vi "Test MQTT-2.3.1-5.vi"(8 "error in (no error)":errorcluster) -> (0 "error out":errorcluster)   [LabVIEW 2013]
uses:
  <vilib>/LabVIEW Open Source Project/MQTT Control Packets/Control Packets/ControlPacket/QualityOfService -- enum.ctl
  <vilib>/LabVIEW Open Source Project/MQTT Control Packets/Control Packets/ControlPacket/ControlPacket.lvclass/ControlPacket.ctl
  <vilib>/addons/_JKI Toolkits/Caraya/classes/Test/Test.lvclass
  <vilib>/addons/_JKI Toolkits/Caraya/classes/Assert/Assert.lvclass
  <vilib>/LabVIEW Open Source Project/MQTT Control Packets/Control Packets/PUBLISH/PUBLISH.lvclass
  <vilib>/LabVIEW Open Source Project/MQTT Control Packets/Control Packets/ControlPacket/ControlPacket.lvclass
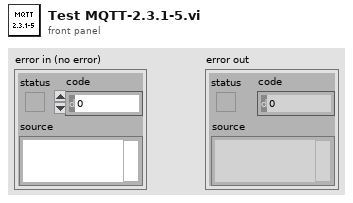
[diagram p1: front panel]
types:
  T1 = typedef "MQTT_Control_Packets.lvlib/ControlPacket.lvclass/QualityOfService -- enum.ctl" = enum16{"0 (At Most Once)", "1 (At Least Once)", "2 (Exactly Once)"}
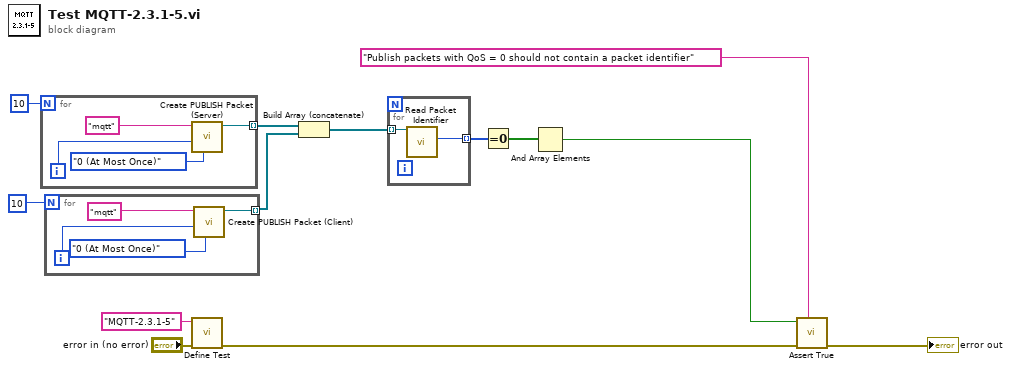
[diagram p0: block diagram]
diagram:
  n1 = for {
    N: 10 -> [_]
    tunnel: [w15] -> w8 mode=indexing
    i -> [w14]
    n2 = call <vilib>:"Create PUBLISH Packet (Server).vi"("QoS"=QualityOfService_--_enum."0 (At Most Once)", "Packet ID (empty: generate new)"=w14, "Topic Name"="mqtt") -> ("PUBLISH"=w15:refnum<class "PUBLISH.lvclass">)  [unwired: 6 in, 2 out]
  }
  n3 = for {
    N: 10 -> [_]
    tunnel: [w19] -> w7 mode=indexing
    i -> [w18]
    n4 = call <vilib>:"Create PUBLISH Packet (Client).vi"("QoS"=QualityOfService_--_enum."0 (At Most Once)", "Packet ID (empty: generate new)"=w18, "Topic Name"="mqtt") -> ("PUBLISH"=w19:refnum<class "PUBLISH.lvclass">)  [unwired: 6 in, 2 out]
  }
  n5 = call <vilib>:"Define Test.vi"("error in (no error)"="error in (no error)", "Label (VI Title)"="MQTT-2.3.1-5") -> ("error out"=w4:errorcluster)  [unwired: 9 in]
  n6 = Build Array (concatenate)(w8, w7) -> (w6:refnum<class "PUBLISH.lvclass">[])
  n7 = for {
    tunnel: w6 -> [w23] mode=indexing
    tunnel: [w22] -> w2 mode=indexing
    n8 = call <vilib>:"Read Packet Identifier.vi"("ControlPacket in"=w23) -> ("Packet Identifier"=w22:u16)  [unwired: 9 in, 1 out]
  }
  n9 = Equal To 0?(x=w2) -> (x = 0?=w1:bool[])
  n10 = And Array Elements(Boolean array=w1) -> (logical AND=w5:bool)
  n11 = call <vilib>:"Assert True.vi"("Label"="Publish packets with QoS = 0 should not contain a packet identifier", "error in (no error)"=w4, "True?"=w5) -> ("error out"=→"error out":errorcluster)  [unwired: 8 in]
